vi "UTIL EMG Filter.vi"(8 "init/cont (init:F)":bool, 10 "Preamp Gain":dbl(ring) items=["10X"=10.0, "100X"=100.0], 11 "EMG In":waveform(dbl)) -> (1 "EMG Power":dbl format="%0.2f", 3 "Filtered EMG Out":waveform(dbl))   [LabVIEW 2017]
doc: "This VI applies a BandPass Butterworth filter to the input EMG Waveform using predetermined filter coefficients from MATLAB. It returns the Filtered EMG (80-100Hz) and the 1-s power r.m.s. power in the 80-100Hz band A notch filter at 60 Hz is also applied prior to the band filters.\n\nInputs:\n EMG In Waveform\n Preamp Gain DBL\n Init/Cont Boolean\nOutputs:\n Filtered EMG Out Waveform\n EMG Power DBL\n Error Out"
uses:
  <vilib>/Analysis/baseanly.llb/Mean (DBL).vi
  <vilib>/Analysis/3filter.llb/IIR Filter (DBL).vi
  <vilib>/Analysis/NI_AALBase.lvlib
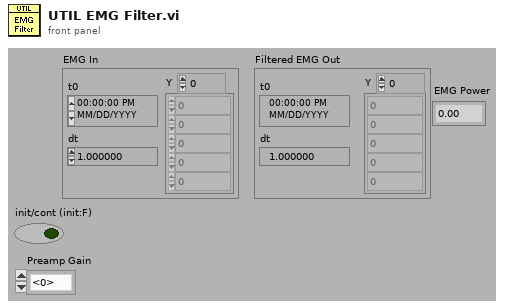
[diagram p1: front panel]
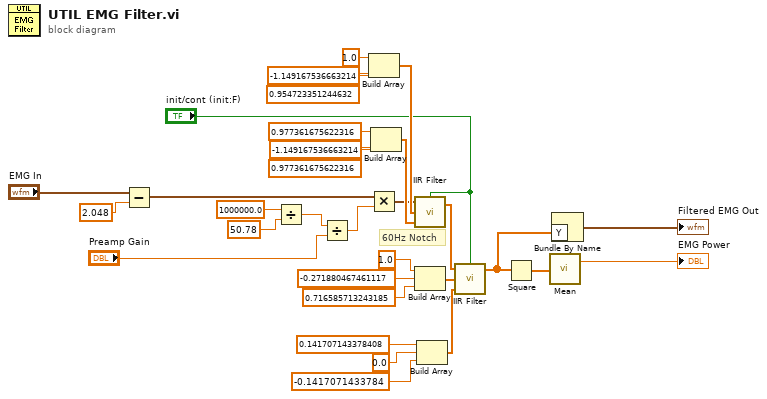
[diagram p0: block diagram]
diagram:
  # "60Hz Notch"
  n1 = Subtract(x="EMG In", y=2.048) -> (x-y=w7:waveform(dbl))
  n2 = Divide(x=1000000.0, y=50.78) -> (x/y=w3:dbl)
  n3 = Divide(x=w3, y="Preamp Gain") -> (x/y=w1:dbl)
  n4 = Build Array(1.0 ("element"), -1.149167536663214 ("element"), 0.954723351244632 ("element")) -> (w24:dbl[])
  n5 = Multiply(x=w7, y=w1) -> (x*y=w9:waveform(dbl))
  n6 = Build Array(0.977361675622316 ("element"), -1.149167536663214 ("element"), 0.977361675622316 ("element")) -> (w23:dbl[])
  n7 = call-poly <vilib>:"IIR Filter.vi"("init/cont (init:F)"="init/cont (init:F)", "Forward Coefficients"=w23, "Reverse Coefficients"=w24, "X"=w9) -> ("Filtered X"=w22:dbl[])  [unwired: 1 out]
  n8 = Build Array(1.0 ("element"), -0.271880467461117 ("element"), 0.716585713243185 ("element")) -> (w14:dbl[])
  n9 = Build Array(0.141707143378408 ("element"), 0.0 ("element"), -0.1417071433784 ("element")) -> (w13:dbl[])
  n10 = call-poly <vilib>:"IIR Filter.vi"("init/cont (init:F)"="init/cont (init:F)", "Forward Coefficients"=w13, "Reverse Coefficients"=w14, "X"=w22) -> ("Filtered X"=w12:dbl[])  [unwired: 1 out]
  n11 = Square(x=w12) -> (x^2=w31:dbl[])
  n12 = call-poly <vilib>:"Mean.vi"("X"=w31) -> ("mean"=→"EMG Power":dbl)  [unwired: 1 out]
  n13 = Bundle By Name("Y"=w12) -> (→"Filtered EMG Out":waveform(dbl))  [unwired: 1 in]
